vi "Fpga_v2.vi"() -> ()   [LabVIEW 2015]
uses:
  <vilib>/rvi/Emulation/niFpgaGetClockAttributes.vi
  <vilib>/rvi/Emulation/niFpgaSctlEmulationGetInTimedLoop.vi
  <vilib>/rvi/Emulation/niFpgaEmulationReportErrorSimple.vi
  <vilib>/rvi/eio/common/nirviEmuTemplateMethod_errors.vi
  <vilib>/rvi/Emulation/niFpgaCriticalErrorInLSC.vi
  <vilib>/rvi/interface/RandomDataEmulation/niFpgaRandomDataHandleErrors.vi
  <vilib>/eio/EIONode/EIONode.xnode
  <vilib>/rvi/DataTransferAndStorage/Container/XNode/niFpgaContainer.xnode
  <vilib>/rvi/interface/RandomDataEmulation/nirviRandomDataFpgaReadWriteTemplate.vi
panel:
  out "x-y":u32
  in  "stop":bool
  out "Mod2/DIO6":bool
  out "Timed Out?":bool
  in  "datachanel":bool
  in  "Data write ON/OFF":bool
  in  "Mod4/AO0 2":i16
  out "Mod3/AI0 2":fxp<+/-,16,5>
  out "Boolean 2":bool
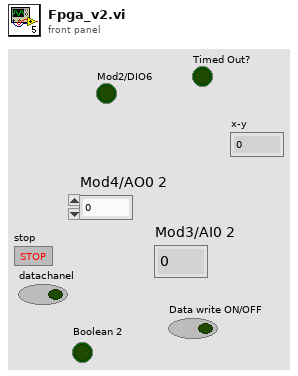
[diagram p1: front panel]
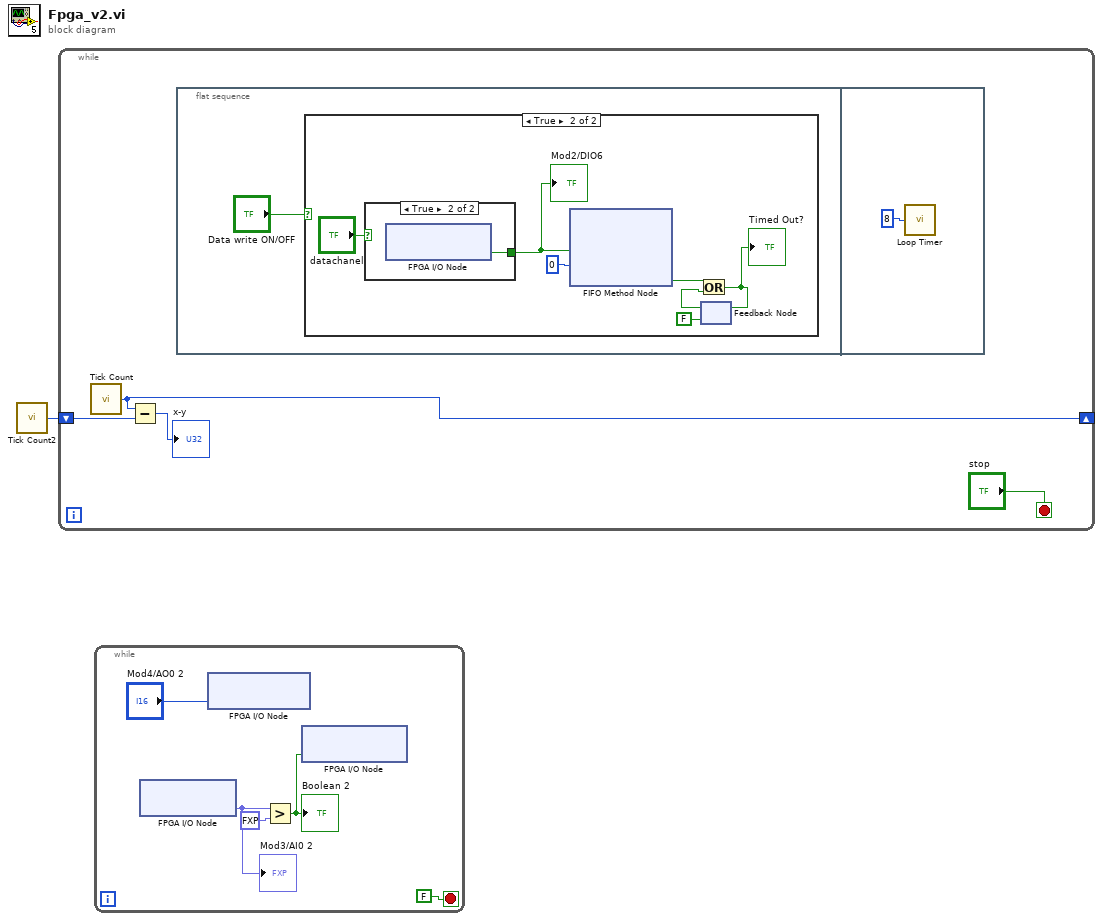
[diagram p0: block diagram]
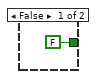
[diagram p3: hidden frame]
diagram:
  n1 = call "Tick Count2"() -> ("Tick Count(Ticks)"=w1:u32)
  n2 = while {
    shift-right: [w5] -> _
    shift-left: w1 -> [w4]
    stop <- "stop" stop-if-true
    n3 = call "Tick Count"() -> ("Tick Count(Ticks)"=w5:u32)
    n4 = Subtract(x=w5, y=w4) -> (x-y=→"x-y":u32)
    n5 = flat-sequence {
      frame #0 {
        n6 = case shown="True" "Data write ON/OFF" {
          frame False {
          }
          frame True {
            n7 = case shown="True" "datachanel" {
              tunnel: [FALSE ("Mod2/DIO6") w15] -> w13
              frame False {
              }
              frame True {
                n8 = xnode "FPGA I/O Node"() -> ("Mod2/DIO6"=w15:bool)  [unwired: 1 in, 1 out]
              }
            }
            "Mod2/DIO6" <- w13
            n9 = xnode ("FIFO Method Node")("Element"=w13, "Timeout"=0) -> ("Timed Out?"=w10:bool)  [unwired: 1 in, 1 out]
            n10 = feedback #1(FALSE) -> (w9:bool)
            n11 = Or(x=w10, y=w9) -> (x .or. y?=w7:bool)
            "Timed Out?" <- w7
            n12 = feedback-in #1(w7) -> ()
          }
        }
      }
      frame #1 {
        n13 = call "Loop Timer"("Count(Ticks)"=u32 8) -> ()  [unwired: 1 out]
      }
    }
  }
  n14 = while {
    stop <- FALSE stop-if-true
    n15 = xnode "FPGA I/O Node"() -> ("Mod3/AI0"=w19:fxp<+/-,16,5>)  [unwired: 1 in, 1 out]
    "Mod3/AI0 2" <- w19
    n16 = xnode "FPGA I/O Node"("Mod4/AO0"="Mod4/AO0 2") -> ()  [unwired: 1 in, 1 out]
    n17 = Greater?(x=w19, y=fxp<+/-,16,5> 2.0) -> (0:w21:bool)
    "Boolean 2" <- w21
    n18 = xnode "FPGA I/O Node"("Mod2/DIO0"=w21) -> ()  [unwired: 1 in, 1 out]
  }
